vi "Simulate_kernal_server.vi"(0 "Board type":T2=enum."Local ADAM", 1 "interval scanning":bool, 2 "Client Time":dbl, 5 "No of samples+extra":i32=128 min=0 step=1, 7 "Trigger mode":T1, 9 "output polarity":u16(ring)=1 items=["do not change", "positive", "negative"], 11 "Ch & spans":T3[](array[typedef]) {"low limit (-10V)" format="%.3f"; "high limit (10V)" format="%.3f"}, 12 "Actual Sampling rate (Hz)":dbl=1000.0 format="%.2f", 13 "Local Client?":bool, 14 "Current Block No":i32) -> (4 "I16 data":i16[][](array[numeric]), 6 "Block Timings":T4={"Started"=0.0, "Ended"=0.0, "Analogue Frequency Hz"=1000.0} {"Analogue Frequency Hz" format="%.2f"}, 10 "group channel settings":T5(array[cluster]) {"scale offset" format="%.2f"; "scale multiplier" format="%.2f"; "gain" format="%.2f"; "range" format="%.2f"; "lower input limits" format="%.2f"; "upper input limits" format="%.2f"}, 15 "error out":errorcluster)   [LabVIEW 2010]
uses:
  Controls/Block_start_and_end.ctl
  Controls/Ch_and_Spans.ctl
  Controls/Board_Types.ctl
  Controls/Trigger_Mode.ctl
  <vilib>/Analysis/NI_AALBase.lvlib
panel:
  in  "Random?":bool
  in  "Average Value":dbl
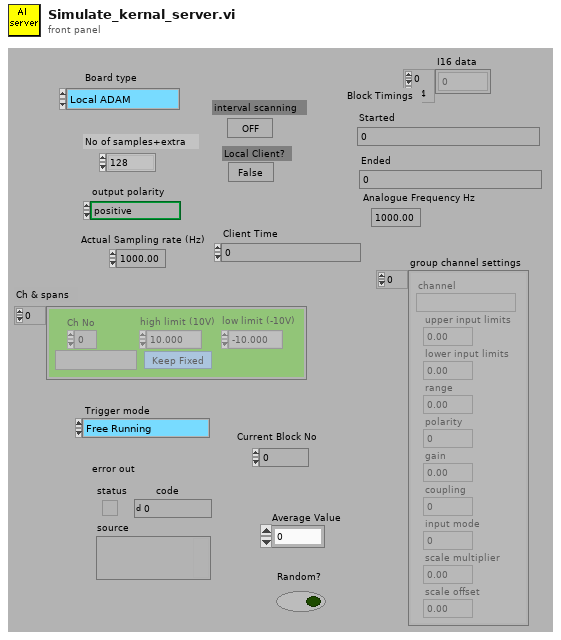
[diagram p1: front panel]
types:
  T1 = typedef "Trigger_Mode.ctl" = enum16{"Free Running", "Start on Trigger", "Trigger Every Block", "Trigger Every Sample"}
  T2 = typedef "Board_Types.ctl" = enum16{"Simulate", "Local ADAM", "Server ADAM", "NI-DAQmx", "NI-DAQmxBase", "ADC488", "DT LV-link"}
  T3 = typedef "Ch_and_Spans.ctl" = cluster{"high limit (10V)":sgl, "low limit (-10V)":sgl, "Ch No":i16, "Var name":string, "Use Latest Calib":bool}
  T4 = typedef "Block_start_and_end.ctl" = cluster{"Started":dbl, "Ended":dbl, "Analogue Frequency Hz":dbl}
  T5 = cluster{"channel":string, "upper input limits":sgl, "lower input limits":sgl, "range":sgl, "polarity":u16, "gain":sgl, "coupling":u16, "input mode":u16, "scale multiplier":dbl, "scale offset":dbl}[]
  T6 = cluster{"channel":string, "upper input limits":sgl, "lower input limits":sgl, "range":sgl, "polarity":u16, "gain":sgl, "coupling":u16, "input mode":u16, "scale multiplier":dbl, "scale offset":dbl}
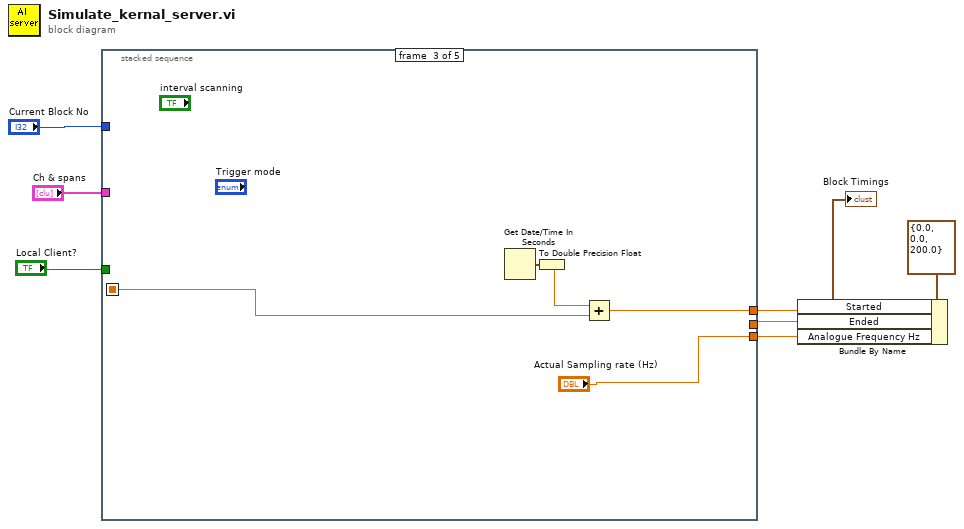
[diagram p0: block diagram]
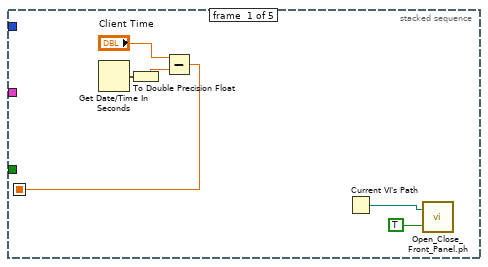
[diagram p2: hidden frame]
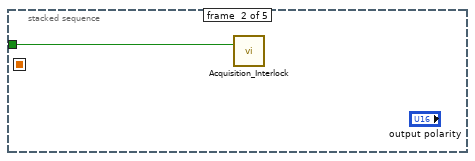
[diagram p3: hidden frame]
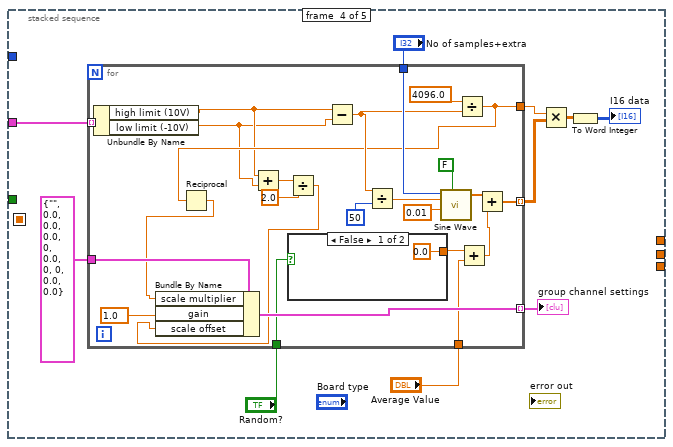
[diagram p4: hidden frame]
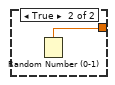
[diagram p5: hidden frame]
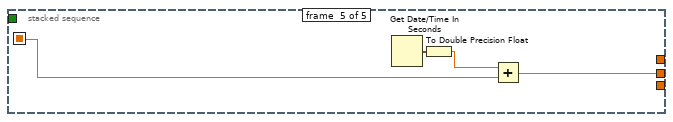
[diagram p6: hidden frame]
diagram:
  n1 = stacked-sequence {
    seq-local: [w12 _ _ _ _] -> [_ _ w18 _ w59]
    tunnel: [_ _ w19 _ _] -> w6
    tunnel: [_ _ _ _ w58] -> w5
    tunnel: "Local Client?" -> [_ w15 _ _ _]
    tunnel: "Ch & spans" -> [_ _ _ w30 _]
    tunnel: "Current Block No" -> [_ _ _ _ _]
    tunnel: [_ _ "Actual Sampling rate (Hz)" _ _] -> w1
    frame #0 {
      n2 = Get Date/Time In Seconds() -> (seconds since 1Jan1904=w11:timestamp)
      n3 = To Double Precision Float(number=w11) -> (double precision float=w13:dbl)
      n4 = Subtract(x="Client Time", y=w13) -> (x-y=w12:dbl)
      n5 = Current VI's Path() -> (path=w10:path)
      n6 = call "Open_Close_Front_Panel.ph.vi"("Front Panel Window:Open"=TRUE, "VI path"=w10) -> ()  [unwired: 2 out]
    }
    frame #1 {
      n7 = call "Acquisition_Interlock.vi"("Local Control"=w15) -> ()
    }
    frame #2 {
      n8 = Get Date/Time In Seconds() -> (seconds since 1Jan1904=w17:timestamp)
      n9 = To Double Precision Float(number=w17) -> (double precision float=w20:dbl)
      n10 = Add(x=w20, y=w18) -> (x+y=w19:dbl)
    }
    frame #3 {
      n11 = for {
        tunnel: [w42] -> w28 mode=indexing
        tunnel: "No of samples+extra" -> [w43]
        tunnel: [w40] -> w27
        tunnel: T6 {"channel"="", "upper input limits"=0.0, "lower input limits"=0.0, "range"=0.0, "polarity"=0, "gain"=0.0, "coupling"=0, "input mode"=0, "scale multiplier"=0.0, "scale offset"=0.0} -> [w48]
        tunnel: [w46] -> w24 mode=indexing
        tunnel: w30 -> [w45] mode=indexing
        tunnel: "Random?" -> [w44]
        tunnel: "Average Value" -> [w36]
        n12 = Unbundle By Name(w45) -> ("high limit (10V)"=w35:sgl, "low limit (-10V)"=w34:sgl)
        n13 = Add(x=w35, y=w34) -> (x+y=w33:sgl)
        n14 = Divide(x=w33, y=sgl 2.0) -> (x/y=w31:sgl)
        n15 = case shown="False" w44 {
          tunnel: [0.0 ("number: 0 to 1") w56] -> w38
          frame False {
          }
          frame True {
            n16 = Random Number (0-1)() -> (number: 0 to 1=w56:dbl)
          }
        }
        n17 = Subtract(x=w35, y=w34) -> (x-y=w41:sgl)
        n18 = Divide(x=w41, y=50) -> (x/y=w50:sgl)
        n19 = call <vilib>:"Sine Wave.vi"("samples"=w43, "amplitude"=w50, "frequency"=0.01 ("f"), "reset phase"=FALSE) -> ("sine wave"=w53:dbl[])  [unwired: 1 in, 2 out]
        n20 = Divide(x=4096.0, y=w41) -> (x/y=w40:dbl)
        n21 = Reciprocal(x=w40) -> (1/x=w39:dbl)
        n22 = Bundle By Name(cluster=w48, "scale multiplier"=w39, "gain"=sgl 1.0 ("Bundle Element"), "scale offset"=w31) -> (w46:T6)
        n23 = Add(x=w38, y=w36) -> (x+y=w37:dbl)
        n24 = Add(x=w53, y=w37) -> (x+y=w42:dbl[])
      }
      "group channel settings" <- w24
      n25 = Multiply(x=w27, y=w28) -> (x*y=w26:dbl[][])
      n26 = To Word Integer(number=w26) -> (16bit integer=→"I16 data":i16[][])
    }
    frame #4 {
      n27 = Get Date/Time In Seconds() -> (seconds since 1Jan1904=w57:timestamp)
      n28 = To Double Precision Float(number=w57) -> (double precision float=w60:dbl)
      n29 = Add(x=w60, y=w59) -> (x+y=w58:dbl)
    }
  }
  n30 = Bundle By Name(cluster=T4 {"Started"=0.0, "Ended"=0.0, "Analogue Frequency Hz"=200.0} ("Block Timings"), "Started"=w6, "Ended"=w5, "Analogue Frequency Hz"=w1) -> (→"Block Timings":T4)
